vi "Query WriteIFile.vi"(8 "error in (no error)":errorcluster, 10 "State":enum16{"Open", "Write", "Close"}(ring), 11 "String":string) -> (0 "error out":errorcluster)   [LabVIEW 2020]
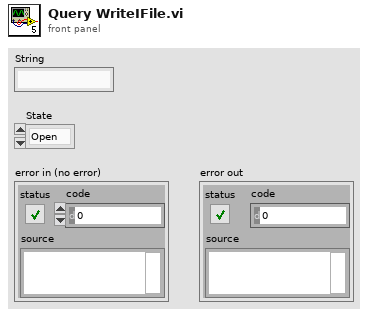
[diagram p1: front panel]
types:
  T1 = enum16{"open", "replace", "create", "open or create", "replace or create", "replace or create with confirmation"}
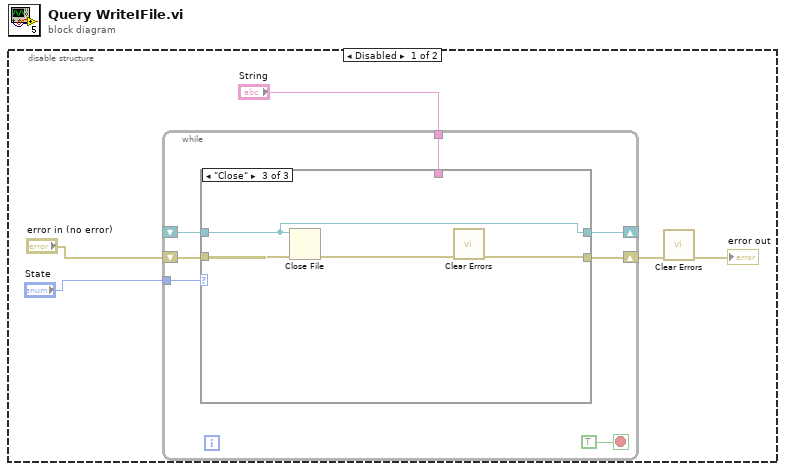
[diagram p0: block diagram]
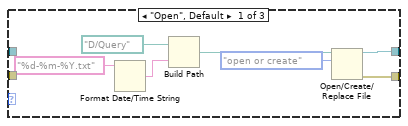
[diagram p2: hidden frame]
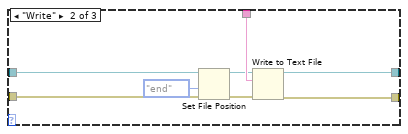
[diagram p3: hidden frame]
diagram:
  n1 = disable-structure shown="Disabled" {
    frame Disabled {
      n2 = while {
        tunnel: "String" -> [w10]
        tunnel: "State" -> [w7]
        shift-right: [w12] -> _
        shift-left: _ -> [w9]
        shift-right: [w11] -> w4
        shift-left: "error in (no error)" -> [w8]
        stop <- TRUE stop-if-true
        n3 = case shown="\"Close\"" w7 {
          tunnel: [w14 w27 w28] -> w12
          tunnel: [w13 w26 w29] -> w11
          tunnel: w10 -> [_ w25 _]
          tunnel: w9 -> [_ w24 w28]
          tunnel: w8 -> [_ w22 w31]
          frame "Open", Default {
            n4 = Format Date/Time String(time format string (%c)="%d-%m-%Y.txt") -> (date/time string=w18:string)  [unwired: 2 in]
            n5 = Build Path(base path=path "D:/Query" ("file (use dialog)"), name or relative path=w18) -> (appended path=w17:path)
            n6 = Open/Create/Replace File(file path (use dialog)=w17, operation (0:open)=T1."open or create") -> (refnum out=w14:refnum<file>, error out=w13:errorcluster)  [unwired: 4 in, 1 out]
          }
          frame "Write" {
            n7 = Set File Position(refnum=w24, from (0:start)=enum16{"start", "end", "current"}."end", error in=w22) -> (refnum out=w23:refnum<file>, error out=w21:errorcluster)  [unwired: 1 in]
            n8 = Write to Text File(file (use dialog)=w23, text=w25, error in=w21) -> (refnum out=w27:refnum<file>, error out=w26:errorcluster)  [unwired: 1 in, 1 out]
          }
          frame "Close" {
            n9 = Close File(refnum=w28, error in=w31) -> (error out=w30:errorcluster)  [unwired: 1 out]
            n10 = call <vilib>:"Clear Errors.vi"("error in (no error)"=w30) -> ("error out"=w29:errorcluster)  [unwired: 5 in, 1 out]
          }
        }
      }
      n11 = call <vilib>:"Clear Errors.vi"("error in (no error)"=w4) -> ("error out"=→"error out":errorcluster)  [unwired: 5 in, 1 out]
    }
    frame Enabled {
    }
  }
